vi "FindAvg.vi"(4 "Main Digitizer":T1=enum."NI Digitizer", 5 "ID":refnum<k15>, 6 "voltage range in":T2, 7 "rf points per line":u16, 8 "Acqiris ID":i32) -> (0 "Vpp":dbl format="%.2f", 1 "Vmin":dbl format="%.2f", 2 "voltage range out":T2, 3 "Vmax":dbl format="%.2f")   [LabVIEW 2022 SP3]
uses:
  ScanningControl/Digitizers/-DigitizerRoutines/Digitizer.ctl
  <vilib>/Analysis/baseanly.llb/Mean (DBL).vi
  <instrlib>/niScope/Acquire/Fetch/niScope Multi Fetch.vi
  <instrlib>/Acqiris Dx/Acqiris Dx.lvlib
  <vilib>/Analysis/NI_AALBase.lvlib
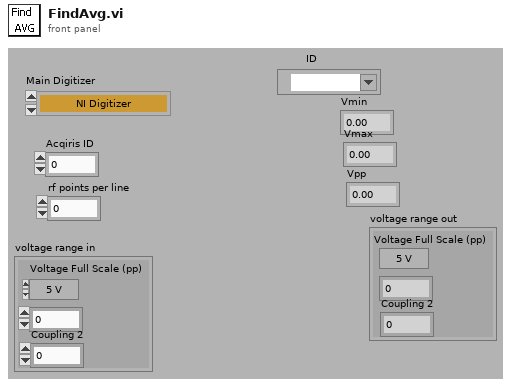
[diagram p1: front panel]
types:
  T1 = typedef "Digitizer.ctl" = enum16{"Acqiris Digitizer", "NI Digitizer", "LeCroy", "GaGe", "AlazarTech", "No Digitizer", "Teledyne"}
  T2 = cluster{"Voltage Full Scale (pp)":u16, i32, "Coupling 2":u16}
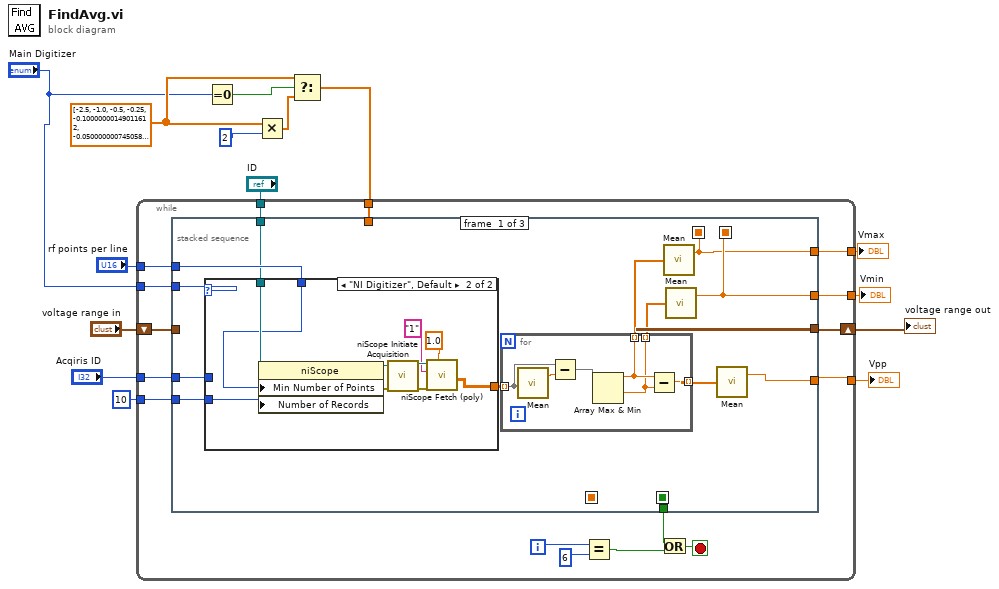
[diagram p0: block diagram]
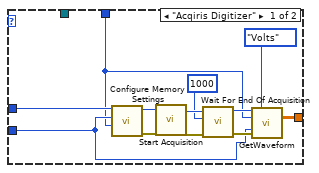
[diagram p2: hidden frame]
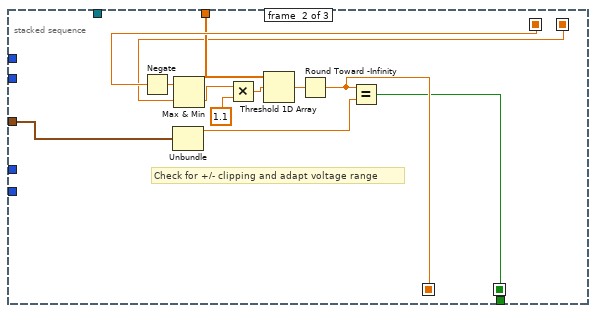
[diagram p3: hidden frame]
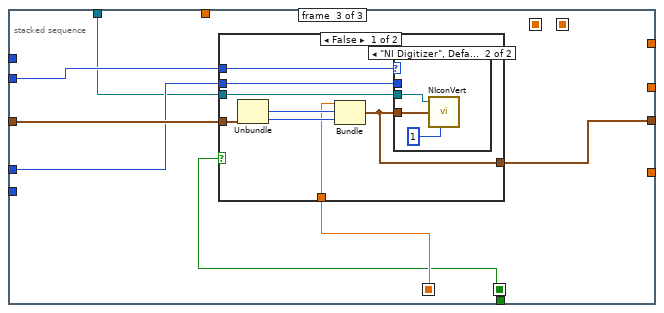
[diagram p4: hidden frame]
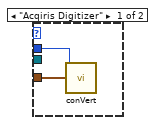
[diagram p5: hidden frame]
diagram:
  w4 = sgl[] [-2.5, -1.0, -0.5, -0.25, -0.1, -0.05, -0.025, 0.0]
  n1 = Equal To 0?(x="Main Digitizer") -> (x = 0?=w3:bool)
  n2 = Multiply(x=w4, y=2) -> (x*y=w6:sgl[])
  n3 = Select(t=w4, s=w3, f=w6) -> (s? t:f=w2:sgl[])
  n4 = while {
    tunnel: [w31] -> w12
    tunnel: "Acqiris ID" -> [w30]
    tunnel: "rf points per line" -> [w29]
    tunnel: [w28] -> w14
    tunnel: [w27] -> w15
    shift-right: [w25] -> w10
    shift-left: "voltage range in" -> [w26]
    tunnel: w2 -> [w24]
    tunnel: 10 -> [w18]
    tunnel: "Main Digitizer" -> [w17]
    tunnel: "ID" -> [w16]
    i -> [w23]
    stop <- w19 stop-if-true
    n5 = stacked-sequence {
      seq-local: [w35 _ _] -> [_ w83 _]
      seq-local: [w41 _ _] -> [_ w79 _]
      seq-local: [_ w72 _] -> [_ _ w86]
      seq-local: [_ w80 _] -> [_ _ w88]
      tunnel: [w43 _ _] -> w31
      tunnel: w30 -> [w42 _ w87]
      tunnel: w29 -> [w34 _ _]
      tunnel: [w35 _ _] -> w28
      tunnel: [w41 _ _] -> w27
      tunnel: w26 -> [_ w81 w90]
      tunnel: [_ _ w89] -> w25
      tunnel: w24 -> [_ w82 _]
      tunnel: [_ w72 _] -> w20
      tunnel: w18 -> [w40 _ _]
      tunnel: w17 -> [w33 _ w85]
      tunnel: w16 -> [w32 _ w84]
      frame #0 {
        n6 = case shown="\"NI Digitizer\", Default" w33 {
          tunnel: w42 -> [w55 _]
          tunnel: w40 -> [w46 w57]
          tunnel: [w45 w61] -> w39
          tunnel: w34 -> [w44 w58]
          tunnel: w32 -> [_ w59]
          frame "Acqiris Digitizer" {
            n7 = call <instrlib>:"Configure Memory Settings.vi"("Number of Samples (1000)"=w44, "Number of Segments (1)"=w46, "Instrument ID"=w55) -> ("error out"=w48:errorcluster, "dup Instrument ID"=w47:u32)  [unwired: 1 in, 2 out]
            n8 = call <instrlib>:"Start Acquisition.vi"("error in (no error)"=w48, "Instrument ID"=w47) -> ("error out"=w52:errorcluster, "dup Instrument ID"=w53:u32)  [unwired: 2 in]
            n9 = call <instrlib>:"Wait For End Of Acquisition.vi"("error in (no error)"=w52, "Timeout"=1000, "Instrument ID"=w53) -> ("error out"=w51:errorcluster, "dup Instrument ID"=w50:u32)  [unwired: 3 out]
            n10 = call "GetWaveform.vi"("Acq ID Out"=w50, "Read Mode"=enum32{"ADC", "Volts"}."Volts", "Num Samps"=w44, "Num Segs"=w46, "error in"=w51) -> ("Acquired Waveform SGL"=w45:dbl[][])  [unwired: 1 in, 9 out]
          }
          frame "NI Digitizer", Default {
            n11 = property class="niScope"(reference=w59, "Min Number of Points"=w58, "Number of Records"=w57) -> (reference out=w65:refnum<k15>, error out=w62:errorcluster)  [unwired: 1 in]
            n12 = call <instrlib>:"niScope Initiate Acquisition.vi"("instrument handle"=w65, "error in"=w62) -> ("instrument handle out"=w63:refnum<k15>, "error out"=w64:errorcluster)  [unwired: 12 out]
            n13 = call-poly <instrlib>:"niScope Fetch (poly).vi"("timeout"=1.0, "error in"=w64, "channels"="1", "instrument handle"=w63) -> ("wfm"=w61:dbl[][])  [unwired: 1 in, 6 out]
          }
        }
        n14 = for {
          tunnel: w39 -> [w67] mode=indexing
          tunnel: [w71] -> w38 mode=indexing
          tunnel: [w70] -> w37 mode=indexing
          tunnel: [w69] -> w36 mode=indexing
          n15 = call-poly <vilib>:"Mean.vi"("X"=w67) -> ("mean"=w68:dbl)  [unwired: 1 out]
          n16 = Subtract(x=w67, y=w68) -> (x-y=w66:dbl[])
          n17 = Array Max & Min(array=w66) -> (max value=w70:dbl, min value=w69:dbl)  [unwired: 2 out]
          n18 = Subtract(x=w70, y=w69) -> (x-y=w71:dbl)
        }
        n19 = call-poly <vilib>:"Mean.vi"("X"=w37) -> ("mean"=w35:dbl)  [unwired: 1 out]
        n20 = call-poly <vilib>:"Mean.vi"("X"=w36) -> ("mean"=w41:dbl)  [unwired: 1 out]
        n21 = call-poly <vilib>:"Mean.vi"("X"=w38) -> ("mean"=w43:dbl)  [unwired: 1 out]
      }
      frame #1 {
        # "Check for +/- clipping and adapt voltage range"
        n22 = Negate(x=w83) -> (-x=w78:dbl)
        n23 = Unbundle(w81) -> ("Voltage Full Scale (pp)"=w74:sgl)  [unwired: 2 out]
        n24 = Max & Min(x=w78, y=w79) -> (min(x,y)=w76:dbl)  [unwired: 1 out]
        n25 = Multiply(x=w76, y=1.1) -> (x*y=w77:dbl)
        n26 = Threshold 1D Array(2:w77, 3:w82) -> (0:w73:sgl)  [unwired: 1 out]
        n27 = Round Toward -Infinity(1:w73) -> (0:w80:sgl)
        n28 = Equal?(x=w80, y=w74) -> (x = y?=w72:bool)
      }
      frame #2 {
        n29 = case shown="False" w86 {
          tunnel: w87 -> [w96 _]
          tunnel: [w95 w104] -> w89
          tunnel: w90 -> [w94 w104]
          tunnel: w88 -> [w93 _]
          tunnel: w85 -> [w92 _]
          tunnel: w84 -> [w91 _]
          frame False {
            n30 = Unbundle(w94) -> (w98:i32, "Coupling 2"=w97:u16)  [unwired: 1 out]
            n31 = Bundle(w93, w98, "Coupling 2"=w97) -> (w95:cluster{sgl, i32, "Coupling 2":u16})  [unwired: 1 out]
            n32 = case shown="\"NI Digitizer\", Default" w92 {
              tunnel: w96 -> [w100 _]
              tunnel: w95 -> [w99 w103]
              tunnel: w91 -> [_ w102]
              frame "Acqiris Digitizer" {
                n33 = call "conVert.vi"("InstrumentID"=w100, "V scale"=w99) -> ()  [unwired: 2 in, 4 out]
              }
              frame "NI Digitizer", Default {
                n34 = call "NIconVert.vi"("InstrumentID"=w102, "V scale"=w103, "Channel (0)"=1) -> ()  [unwired: 1 in, 4 out]
              }
            }
          }
          frame True {
          }
        }
      }
    }
    n35 = Equal?(x=w23, y=6) -> (x = y?=w21:bool)
    n36 = Or(x=w20, y=w21) -> (x .or. y?=w19:bool)
  }
  "Vmin" <- w15
  "Vmax" <- w14
  "Vpp" <- w12
  "voltage range out" <- w10
